vi "FRCts20_WebMethods_Competition_GET.vi"(6 "query":string, 7 "httpRequestID":u32, 11 "competition":string) -> ()   [LabVIEW 2014]
doc: "<B>GET</B> on the specified <B>competition</B> resource\n\n<B>Default Return:</B> <B>competition</B> information and list of contained divisions\n\n<B>query =</B> info - Returns only <B>competition</B> information\n stats - Returns statistics for <B>competition</B>\n images - Returns .png and .jpeg images for <B>competition</B>\n videos - Returns .wmv videos for <B>competition</B>\n\nhttp://<server address>:<port>/FRCts/competition/<B>competition</B>"
uses:
  <vilib>/wsapi/NI_WebServices.lvlib
  FRCts20_WebMethods.lvlib
  Backend/source/VI Source/FRCts20_Backend_API/FRCts20_Backend_API.lvlib
  Backend/source/VI Source/FRCts20_Backend_API/FRCts20_Backend_API_Command_CompRoot.ctl
  Backend/source/VI Source/FRCts20_Backend_API/FRCts20_Backend_API_Competition.ctl
  Backend/source/VI Source/FRCts20_Backend_API/FRCts20_Backend_API_Stats.vi
  Backend/source/VI Source/FRCts20_Backend_API/FRCts20_Backend_API_Command_Stats.ctl
  Backend/source/VI Source/FRCts20_Backend_API/FRCts20_Backend_API_Stats.ctl
  Backend/source/VI Source/FRCts20_Backend_API/FRCts20_Backend_API_EventRoot.vi
  Backend/source/VI Source/FRCts20_Backend_API/FRCts20_Backend_API_Application.vi
  ESP Engine/source/VI Source/TypeDefs/FRCts20_EspEngine_AdvancedComponents_Bar.ctl
  ESP Engine/source/VI Source/FRCts20_EspEngine.lvlib
  ESP Engine/source/VI Source/TypeDefs/FRCts20_EspEngine_SwUsage_Pie.ctl
  ESP Engine/source/VI Source/TypeDefs/FRCts20_EspEngine_RequestPerHour_Line.ctl
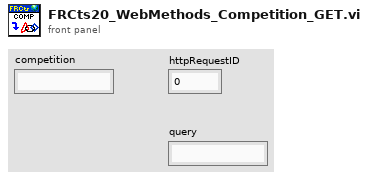
[diagram p1: front panel]
types:
  T1 = typedef "FRCts20_Backend_API.lvlib/FRCts20_Backend_API_Command_CompRoot.ctl" = string
  T2 = typedef "FRCts20_Backend_API.lvlib/FRCts20_Backend_API_Competition.ctl" = cluster{"Name":string, "Start Date":timestamp, "Duration":u8, "Divisions":string[], "APIReturn":string}
  T3 = typedef "FRCts20_Backend_API.lvlib/FRCts20_Backend_API_Stats.ctl" = cluster{"RequestsPerHour":T4, "SW Usage Pies":T5, "Advanced Components":T6, "APIReturn":string}
  T4 = typedef "FRCts20_EspEngine.lvlib/FRCts20_EspEngine_RequestPerHour_Line.ctl" = cluster{"StartDate":cluster{"Year":i32, "Month":i32, "Day":i32}, "Events":cluster{"Location":string, "Requests":i32[]}[]}
  T5 = typedef "FRCts20_EspEngine.lvlib/FRCts20_EspEngine_SwUsage_Pie.ctl" = cluster{"Live Event Location":string, "LabVIEW":dbl, "C++":dbl, "Java":dbl, "Other":dbl, "TotalTeams":i32, "TeamsReporting":i32}[]
  T6 = typedef "FRCts20_EspEngine.lvlib/FRCts20_EspEngine_AdvancedComponents_Bar.ctl" = cluster{"CAN":i32, "Vision":i32, "Kinect":i32}
  T7 = typedef "FRCts20_Backend_API.lvlib/FRCts20_Backend_API_Command_Stats.ctl" = string
  T8 = typedef "FRCts20_Backend_API.lvlib/FRCts20_Backend_API_EventRoot.ctl" = cluster{"Event":cluster{"Event Index":u32, "EventID":u32, "EventSubtype":string, "EventSubtypeID":u32, "DistrictCode":string, "DistrictID":u32, "Event Name":string, "Venue":string, "City":string, "StateProvince":string, "Country":string, "Start Time":timestamp, "End Time":timestamp, "Year":u32, "NumberOfTeams":u32, "URLTeamlist":string, "EventCode":string, "OpenIssues":u8, "IsLive":bool}[], "APIReturn":string}
  T9 = typedef "FRCts20_Backend_API.lvlib/FRCts20_Backend_API_Application.ctl" = cluster{"Revision":string, "APIReturn":string}
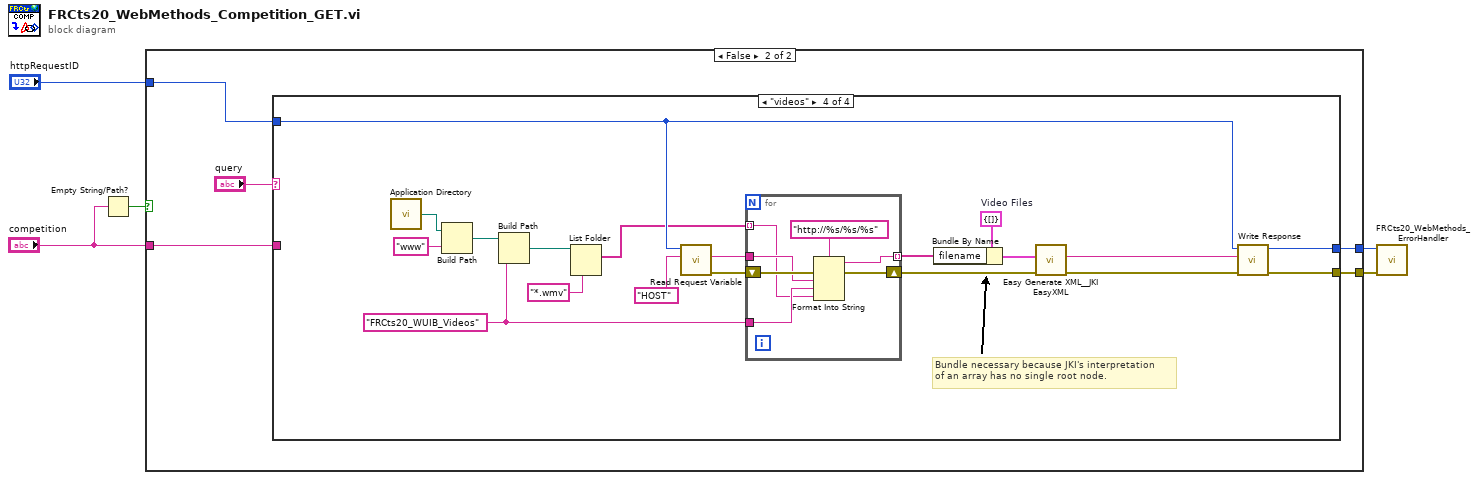
[diagram p0: block diagram]
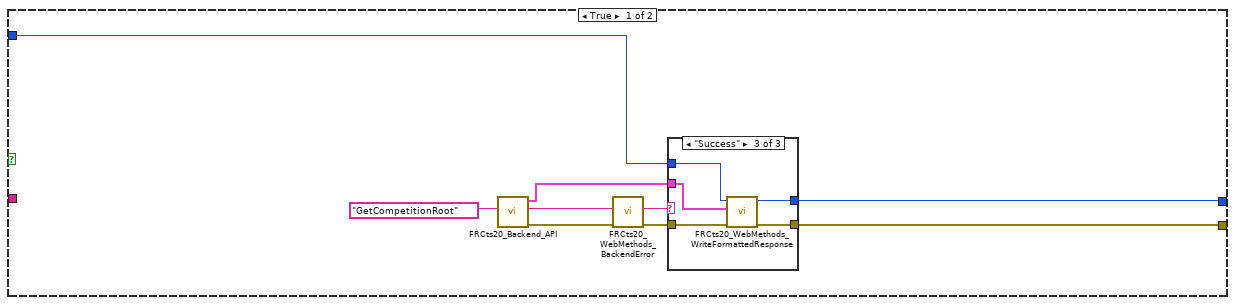
[diagram p2: hidden frame]
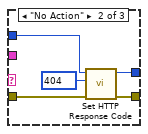
[diagram p4: hidden frame]
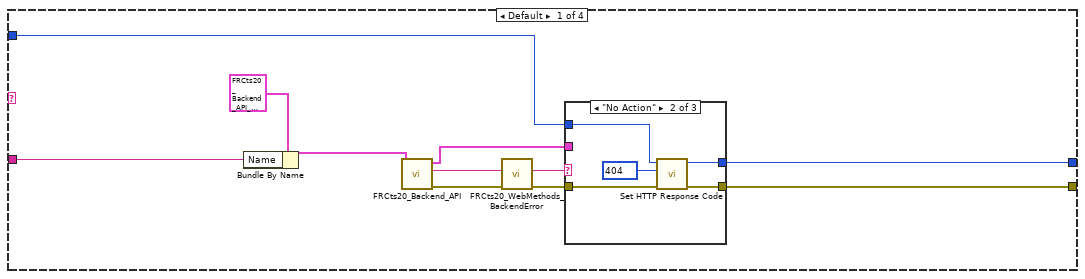
[diagram p5: hidden frame]
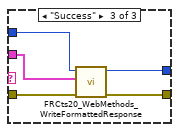
[diagram p7: hidden frame]
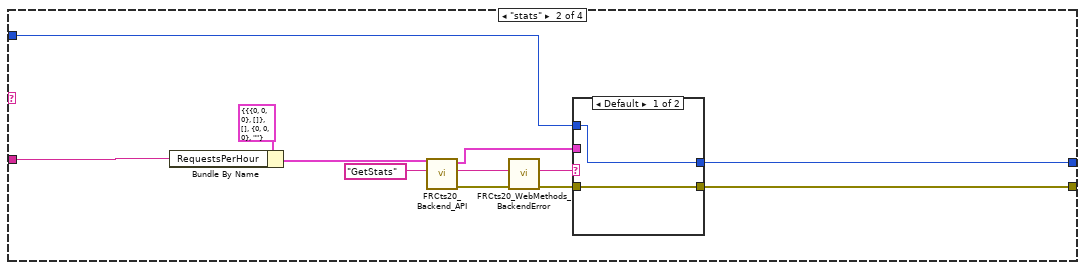
[diagram p8: hidden frame]
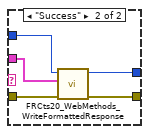
[diagram p9: hidden frame]
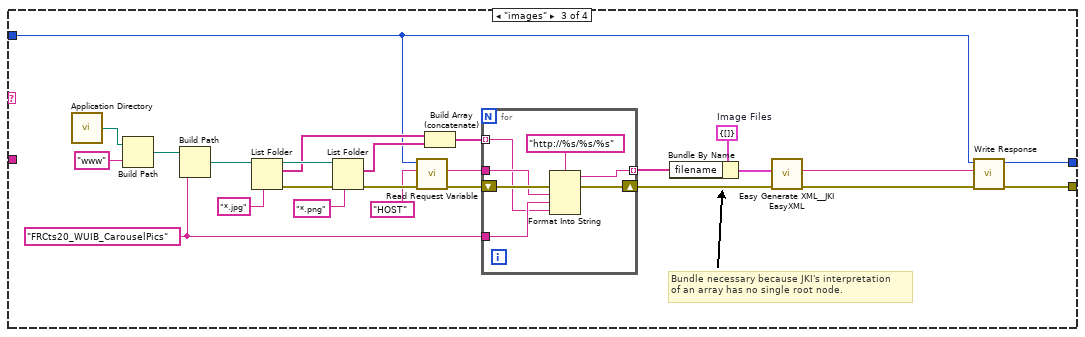
[diagram p10: hidden frame]
diagram:
  n1 = Empty String/Path?(string/path="competition") -> (empty?=w2:bool)
  n2 = case shown="False" w2 {
    tunnel: "httpRequestID" -> [w9 w31]
    tunnel: [w7 w30] -> w4
    tunnel: [w6 w29] -> w3
    tunnel: "competition" -> [_ w27]
    frame True {
      n3 = call-poly "FRCts20_Backend_API.vi"("Message"=T1 "GetCompetitionRoot") -> ("error out"=w13:errorcluster, "Status"=w12:string, "EventRoot Out"=w8:T8)  [unwired: 8 in]
      n4 = call "FRCts20_WebMethods_BackendError.vi"("error in (no error)"=w13, "Status"=w12) -> ("error out"=w10:errorcluster, "Status out"=w11:string)  [unwired: 8 in]
      n5 = case shown="\"Success\"" w11 {
        tunnel: w10 -> [w15 w20 w26]
        tunnel: w9 -> [w16 w19 w25]
        tunnel: w8 -> [_ _ w24]
        tunnel: [w16 w17 w23] -> w6
        tunnel: [w15 w21 w22] -> w7
        frame "Backend Error", Default {
        }
        frame "No Action" {
          w18 = 404 items=["100"=100, "101"=101, "200"=200, "201"=201, "202"=202, "203"=203, "204"=204, "205"=205, "206"=206, "300"=300, "301"=301, "302"=302, "303"=303, "304"=304, "305"=305, "306"=306, "307"=307, "400"=400, "401"=401, "402"=402, "403"=403, "404"=404, "405"=405, "406"=406, "407"=407, "408"=408, "409"=409, "410"=410, "411"=411, "412"=412, "413"=413, "414"=414, "415"=415, "416"=416, "417"=417, "500"=500, "501"=501, "502"=502, "503"=503, "504"=504, "505"=505] ("response code (200)")
          n6 = call <vilib>:"Set HTTP Response Code.vi"("error in (no error)"=w20, "response code (200)"=w18, "httpRequestID"=w19) -> ("error out"=w21:errorcluster, "httpRequestID out"=w17:u32)  [unwired: 7 in]
        }
        frame "Success" {
          n7 = call "FRCts20_WebMethods_WriteFormattedResponse.vi"("error in (no error)"=w26, "Response Cluster"=w24, "httpRequestID"=w25) -> ("error out"=w22:errorcluster, "httpRequestID out"=w23:u32)  [unwired: 7 in]
        }
      }
    }
    frame False {
      n8 = case shown="\"videos\"" "query" {
        tunnel: w31 -> [w35 w60 w82 w115]
        tunnel: [w33 w58 w89 w120] -> w30
        tunnel: [w34 w59 w88 w119] -> w29
        tunnel: w27 -> [w41 w57 _ _]
        frame Default {
          n9 = Bundle By Name(cluster=T2 {"Name"="", "Start Date"=timestamp(0 s since 1904-01-01), "Duration"=0, "Divisions"=[], "APIReturn"=""} ("Competition"), "Name"=w41) -> (w32:T2)
          n10 = call-poly "FRCts20_Backend_API.vi"(11:w32) -> ("error out"=w40:errorcluster, "Status"=w39:string, "Application"=w36:T9)  [unwired: 8 in]
          n11 = call "FRCts20_WebMethods_BackendError.vi"("error in (no error)"=w40, "Status"=w39) -> ("error out"=w37:errorcluster, "Status out"=w38:string)  [unwired: 8 in]
          n12 = case shown="\"No Action\"" w38 {
            tunnel: w37 -> [w43 w45 w54]
            tunnel: w36 -> [_ _ w53]
            tunnel: w35 -> [w44 w47 w52]
            tunnel: [w44 w48 w51] -> w34
            tunnel: [w43 w49 w50] -> w33
            frame "Backend Error", Default {
            }
            frame "No Action" {
              w46 = 404 items=["100"=100, "101"=101, "200"=200, "201"=201, "202"=202, "203"=203, "204"=204, "205"=205, "206"=206, "300"=300, "301"=301, "302"=302, "303"=303, "304"=304, "305"=305, "306"=306, "307"=307, "400"=400, "401"=401, "402"=402, "403"=403, "404"=404, "405"=405, "406"=406, "407"=407, "408"=408, "409"=409, "410"=410, "411"=411, "412"=412, "413"=413, "414"=414, "415"=415, "416"=416, "417"=417, "500"=500, "501"=501, "502"=502, "503"=503, "504"=504, "505"=505] ("response code (200)")
              n13 = call <vilib>:"Set HTTP Response Code.vi"("error in (no error)"=w45, "response code (200)"=w46, "httpRequestID"=w47) -> ("error out"=w49:errorcluster, "httpRequestID out"=w48:u32)  [unwired: 7 in]
            }
            frame "Success" {
              n14 = call "FRCts20_WebMethods_WriteFormattedResponse.vi"("error in (no error)"=w54, "Response Cluster"=w53, "httpRequestID"=w52) -> ("error out"=w50:errorcluster, "httpRequestID out"=w51:u32)  [unwired: 7 in]
            }
          }
        }
        frame "stats" {
          n15 = Bundle By Name(cluster=T3 {"RequestsPerHour"={"StartDate"={"Year"=0, "Month"=0, "Day"=0}, "Events"=[]}, "SW Usage Pies"=[], "Advanced Components"={"CAN"=0, "Vision"=0, "Kinect"=0}, "APIReturn"=""} ("Statistics"), "RequestsPerHour"=w57) -> (w55:T3)
          n16 = call-poly "FRCts20_Backend_API.vi"("Command"=T7 "GetStats", "Statistics In"=w55) -> ("error out"=w65:errorcluster, "Status"=w64:string, "Statistics Out"=w61:T3)  [unwired: 7 in]
          n17 = call "FRCts20_WebMethods_BackendError.vi"("error in (no error)"=w65, "Status"=w64) -> ("error out"=w62:errorcluster, "Status out"=w63:string)  [unwired: 8 in]
          n18 = case shown="Default" w63 {
            tunnel: w62 -> [w67 w73]
            tunnel: w61 -> [_ w72]
            tunnel: w60 -> [w68 w71]
            tunnel: [w68 w70] -> w59
            tunnel: [w67 w69] -> w58
            frame Default {
            }
            frame "Success" {
              n19 = call "FRCts20_WebMethods_WriteFormattedResponse.vi"("error in (no error)"=w73, "Response Cluster"=w72, "httpRequestID"=w71) -> ("error out"=w69:errorcluster, "httpRequestID out"=w70:u32)  [unwired: 7 in]
            }
          }
        }
        frame "images" {
          w76 = cluster{"filename":string[]} {"filename"=[]}  # Image Files
          w78 = "FRCts20_WUIB_CarouselPics" ("name or relative path")
          # "Bundle necessary because JKI's interpretation \nof an array has no single root node."
          n20 = call <vilib>:"Application Directory.vi"() -> ("Application Directory"=w87:path)
          n21 = Build Path(base path=w87, name or relative path="www") -> (appended path=w86:path)
          n22 = Build Path(base path=w86, name or relative path=w78) -> (appended path=w85:path)
          n23 = List Folder(path=w85, pattern="*.jpg") -> (path out=w96:path, filenames=w93:string[], error out=w95:errorcluster)  [unwired: 2 in, 1 out]
          n24 = List Folder(path=w96, pattern="*.png", error in=w95) -> (filenames=w92:string[], error out=w83:errorcluster)  [unwired: 1 in, 2 out]
          n25 = call <vilib>:"Read Request Variable.vi"("error in (no error)"=w83, "variable name"="HOST", "httpRequestID"=w82) -> ("error out"=w80:errorcluster, "value"=w79:string)  [unwired: 6 in, 1 out]
          n26 = Build Array (concatenate)(w93, w92) -> (w84:string[])
          n27 = for {
            tunnel: w84 -> [w99] mode=indexing
            shift-right: [w105] -> w77
            shift-left: w80 -> [w104]
            tunnel: w79 -> [w101]
            tunnel: w78 -> [w100]
            tunnel: [w103] -> w74 mode=indexing
            n28 = Format Into String(format string="http://%s/%s/%s", error in=w104, w101, w100, w99) -> (resulting string=w103:string, error out=w105:errorcluster)  [unwired: 1 in]
          }
          n29 = Bundle By Name(cluster=w76, "filename"=w74) -> (w75:cluster{"filename":string[]})
          n30 = call <vilib>:"Easy Generate XML__JKI EasyXML.vi"("error in (no error)"=w77, "LabVIEW Data"=w75) -> ("error out"=w90:errorcluster, "XML String"=w91:string)  [unwired: 8 in]
          n31 = call <vilib>:"Write Response.vi"("error in (no error)"=w90, "response string"=w91, "httpRequestID"=w82) -> ("error out"=w89:errorcluster, "httpRequestID out"=w88:u32)  [unwired: 7 in]
        }
        frame "videos" {
          w109 = cluster{"filename":string[]} {"filename"=[]}  # Video Files
          w111 = "FRCts20_WUIB_Videos" ("name or relative path")
          # "Bundle necessary because JKI's interpretation \nof an array has no single root node."
          n32 = call <vilib>:"Application Directory.vi"() -> ("Application Directory"=w118:path)
          n33 = Build Path(base path=w118, name or relative path="www") -> (appended path=w117:path)
          n34 = Build Path(base path=w117, name or relative path=w111) -> (appended path=w116:path)
          n35 = List Folder(path=w116, pattern="*.wmv") -> (filenames=w106:string[])  [unwired: 2 in, 3 out]
          n36 = call <vilib>:"Read Request Variable.vi"("variable name"="HOST", "httpRequestID"=w115) -> ("error out"=w113:errorcluster, "value"=w112:string)  [unwired: 7 in, 1 out]
          n37 = for {
            tunnel: w106 -> [w125] mode=indexing
            shift-right: [w131] -> w110
            shift-left: w113 -> [w130]
            tunnel: w112 -> [w127]
            tunnel: w111 -> [w126]
            tunnel: [w129] -> w107 mode=indexing
            n38 = Format Into String(format string="http://%s/%s/%s", error in=w130, w127, w126, w125) -> (resulting string=w129:string, error out=w131:errorcluster)  [unwired: 1 in]
          }
          n39 = Bundle By Name(cluster=w109, "filename"=w107) -> (w108:cluster{"filename":string[]})
          n40 = call <vilib>:"Easy Generate XML__JKI EasyXML.vi"("error in (no error)"=w110, "LabVIEW Data"=w108) -> ("error out"=w121:errorcluster, "XML String"=w122:string)  [unwired: 8 in]
          n41 = call <vilib>:"Write Response.vi"("error in (no error)"=w121, "response string"=w122, "httpRequestID"=w115) -> ("error out"=w120:errorcluster, "httpRequestID out"=w119:u32)  [unwired: 7 in]
        }
      }
    }
  }
  n42 = call "FRCts20_WebMethods_ErrorHandler.vi"("error in"=w4, "httpRequestID"=w3) -> ()  [unwired: 9 in, 1 out]
